vi "Save Log File.vi"(8 "error in (no error)":errorcluster, 11 "Str Refnum":refnum<vi>) -> (0 "Error out":errorcluster, 3 "UI Settings":T1={"Font"="Consolas", "Font Size"=0, "BG Color"=0, "Text Color"=0, "Debug?"=FALSE})   [LabVIEW 2023, in "VeriStand Console.lvlib"]
uses:
  VeriStand Console.lvlib
  TypeDefs/UI Settings.ctl
  <vilib>/registry/registry.llb/Registry RtKey.ctl
  <vilib>/registry/registry.llb/Registry SAM.ctl
  8dee9384-0adc-4c69-98de-5d373f74b021.vi
panel:
  in  "OK":bool
  in  "Background Color":u32(colorbox)
  in  "Text Color":u32(colorbox)
  in  "Size":string(combo)
  in  "Font":string(combo)
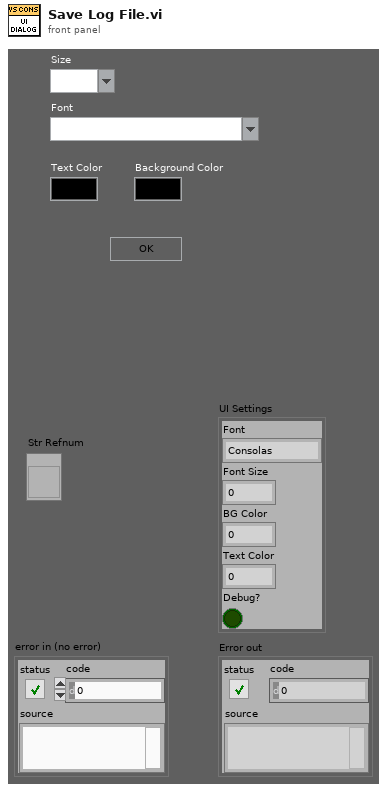
[diagram p1: front panel]
types:
  T1 = typedef "VeriStand Console.lvlib/UI Settings.ctl" = cluster{"Font":string, "Font Size":u32, "BG Color":u32, "Text Color":u32, "Debug?":bool}
  T2 = typedef "Registry SAM.ctl" = enum32{"KEY_QUERY_VALUE", "KEY_SET_VALUE", "KEY_CREATE_SUB_KEY", "KEY_ENUMERATE_SUB_KEYS", "KEY_NOTIFY", "KEY_CREATE_LINK", "KEY_READ", "KEY_WRITE", "KEY_ALL_ACCESS", "KEY_READ | KEY_WRITE"}
  T3 = typedef "Registry RtKey.ctl" = enum32{"HKEY_CLASSES_ROOT", "HKEY_CURRENT_USER", "HKEY_LOCAL_MACHINE", "HKEY_USERS", "HKEY_PERFORMANCE_DATA", "HKEY_CURRENT_CONFIG", "HKEY_DYN_DATA"}
  T4 = typedef "Registry refnum.ctl" = refnum<k1>
  T5 = cluster{"numValues":i32, "maxValueNameLen":i32, "maxValueDataLen":i32}
  T6 = cluster{"value name":string, "value name":string}
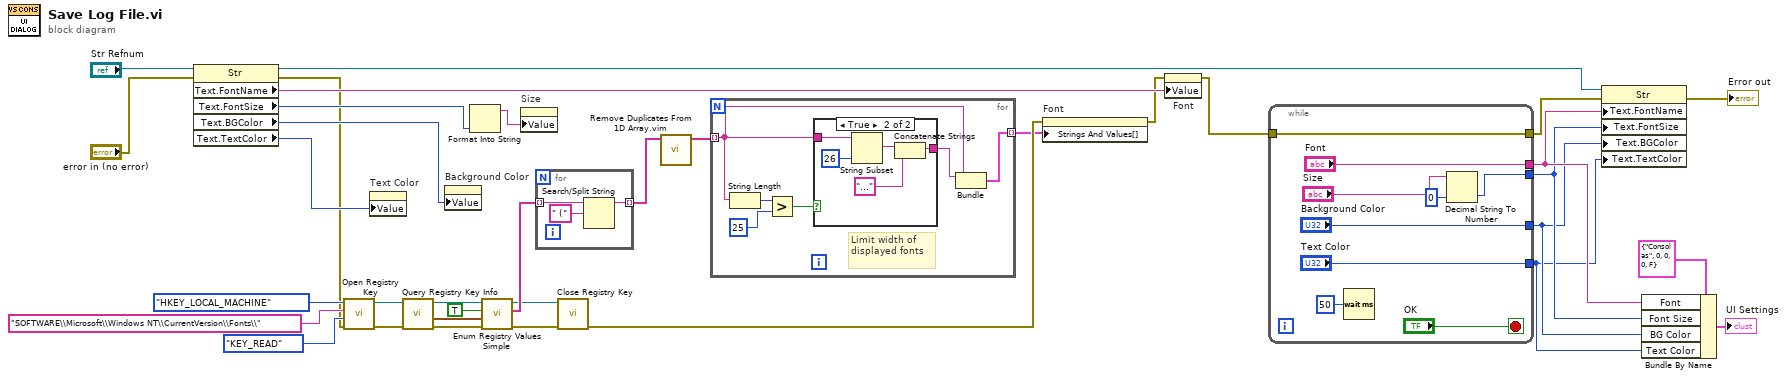
[diagram p0: block diagram]
diagram:
  n1 = property class="Str"(reference="Str Refnum", error in="error in (no error)") -> (reference out=w14:refnum<vi>, error out=w10:errorcluster, "Text.FontName"=w18:string, "Text.FontSize"=w22:u32, "Text.BGColor"=w19:u32, "Text.TextColor"=w20:u32)
  n2 = call <vilib>:"Open Registry Key.vi"("error in (no error)"=w10, "security access mask (KEY_READ | KEY_WRITE)"=Registry_SAM."KEY_READ", "subkey"="SOFTWARE\\Microsoft\\Windows NT\\CurrentVersion\\Fonts\\", "root key (HKEY_LOCAL_MACHINE)"=Registry_RtKey."HKEY_LOCAL_MACHINE") -> ("error out"=w27:errorcluster, "refnum out"=w26:T4)  [unwired: 6 in]
  n3 = property on="Text Color" class="ColBox"("Value"=w20) -> ()  [unwired: 2 in, 2 out]
  n4 = call <vilib>:"Query Registry Key Info.vi"("error in (no error)"=w27, "refnum"=w26) -> ("error out"=w30:errorcluster, "value info"=w33:T5, "refnum out"=w29:T4)  [unwired: 5 in, 2 out]
  n5 = property on="Background Color" class="ColBox"("Value"=w19) -> ()  [unwired: 2 in, 2 out]
  n6 = Format Into String(w22) -> (resulting string=w21:string)  [unwired: 3 in, 1 out]
  n7 = call <vilib>:"Enum Registry Values Simple.vi"("error in (no error)"=w30, "value info"=w33, "retrieve data? (F)"=TRUE, "refnum"=w29) -> ("error out"=w31:errorcluster, "values"=w35:string[], "refnum out"=w32:T4)  [unwired: 2 in, 3 out]
  n8 = property on="Size" class="CmbBox"("Value"=w21) -> ()  [unwired: 2 in, 2 out]
  n9 = for {
    tunnel: w35 -> [w38] mode=indexing
    tunnel: [w36] -> w2 mode=indexing
    n10 = Search/Split String(string=w38, search string/char (-)=" (") -> (substring before match=w36:string)  [unwired: 1 in, 2 out]
  }
  n11 = call <vilib>:"Close Registry Key.vi"("error in (no error)"=w31, "refnum"=w32) -> ("error out"=w15:errorcluster)  [unwired: 5 in]
  n12 = call "Remove Duplicates From 1D Array.vim"("array"=w2) -> ("array with duplicates removed"=w1:string[])  [unwired: 10 in]
  n13 = for {
    tunnel: w1 -> [w42] mode=indexing
    tunnel: [w43] -> w3 mode=indexing
    # "Limit width of displayed fonts"
    n14 = String Length(string=w42) -> (length=w41:i32)
    n15 = Greater?(x=w41, y=25) -> (0:w39:bool)
    n16 = case shown="True" w39 {
      tunnel: [w45 w46] -> w44
      tunnel: w42 -> [w45 w49]
      frame False {
      }
      frame True {
        n17 = String Subset(string=w49, length (rest)=26 ("length (rest)")) -> (substring=w48:string)  [unwired: 1 in]
        n18 = Concatenate Strings(w48, "..." ("string")) -> (w46:string)
      }
    }
    n19 = Bundle("value name"=w44, "value name"=w42) -> (w43:T6)  [unwired: 1 in]
  }
  n20 = property on="Font" class="CmbBox"(error in=w15, "Strings And Values[]"=w3) -> (error out=w17:errorcluster)  [unwired: 1 in, 1 out]
  n21 = property on="Font" class="CmbBox"(error in=w17, "Value"=w18) -> (error out=w16:errorcluster)  [unwired: 1 in, 1 out]
  n22 = while {
    tunnel: w16 -> [w51]
    tunnel: ["Text Color"] -> w5
    tunnel: ["Background Color"] -> w6
    tunnel: [w53] -> w7
    tunnel: ["Font"] -> w8
    tunnel: [w51] -> w13
    stop <- "OK" stop-if-true
    n23 = Wait (ms)(milliseconds to wait=u32 50) -> ()  [unwired: 1 out]
    n24 = Decimal String To Number(string="Size", default (0L)=u32 0 ("default (0 I32)")) -> (number=w53:u32)  [unwired: 1 in, 1 out]
  }
  n25 = property class="Str"(reference=w14, error in=w13, "Text.FontName"=w8, "Text.FontSize"=w7, "Text.BGColor"=w6, "Text.TextColor"=w5) -> (error out=→"Error out":errorcluster)  [unwired: 1 out]
  n26 = Bundle By Name(cluster=T1 {"Font"="Consolas", "Font Size"=0, "BG Color"=0, "Text Color"=0, "Debug?"=FALSE} ("UI Settings"), "Font"=w8, "Font Size"=w7, "BG Color"=w6, "Text Color"=w5) -> (→"UI Settings":T1)
